vi "InMotion.vi"(0 "System no.":i32, 2 "Axes to check":string[](array[string]), 5 "error in (no error)":errorcluster, 9 "With status bit polling?":bool) -> (14 "InMotion":bool, 16 "Motion Error":bool, 19 "error out":errorcluster)   [LabVIEW 2020]
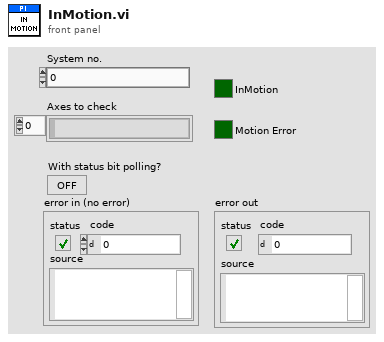
[diagram p1: front panel]
types:
  T1 = typedef "Syntax.ctl" = enum16{"GCS 1.0", "GCS 2.0", "GCS 3.0"}
  T2 = typedef "Status.ctl" = cluster{"Element":string, "Status bits":bool[]}
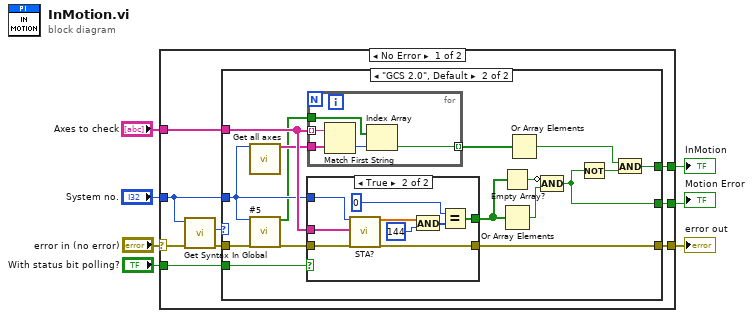
[diagram p0: block diagram]
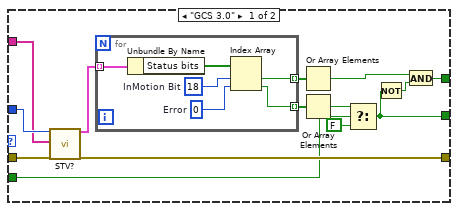
[diagram p2: hidden frame]
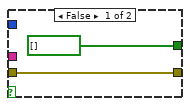
[diagram p3: hidden frame]
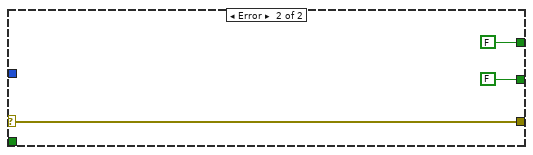
[diagram p4: hidden frame]
diagram:
  n1 = case shown="No Error" "error in (no error)" {
    selector: "error in (no error)" -> [w8 w71]
    tunnel: [w16 FALSE] -> w7
    tunnel: [w15 w71] -> w6
    tunnel: "With status bit polling?" -> [w14 _]
    tunnel: "Axes to check" -> [w13 _]
    tunnel: "System no." -> [w10 _]
    tunnel: [w9 FALSE] -> w2
    frame No Error {
      n2 = call "Get Syntax In Global.vi"("error in"=w8, "System no."=w10) -> ("error out"=w12:errorcluster, "Syntax"=w11:T1)  [unwired: 8 in]
      n3 = case shown="\"GCS 2.0\", Default" w11 {
        tunnel: w10 -> [w30 w47]
        tunnel: w12 -> [w29 w52]
        tunnel: [w28 w50] -> w15
        tunnel: [w19 w38] -> w16
        tunnel: w13 -> [w26 w49]
        tunnel: w14 -> [w21 w48]
        tunnel: [w17 w40] -> w9
        frame "GCS 3.0" {
          n4 = call "STV?.vi"("System no."=w30, "Status Type"=w26, "error in"=w29) -> ("Status Array"=w27:T2[], "error out"=w28:errorcluster)  [unwired: 15 in]
          n5 = for {
            tunnel: w27 -> [w36] mode=indexing
            tunnel: [w33] -> w25 mode=indexing
            tunnel: [w31] -> w23 mode=indexing
            w32 = 0  # Error
            w34 = 18  # InMotion Bit
            n6 = Unbundle By Name(w36) -> ("Status bits"=w35:bool[])
            n7 = Index Array(array=w35, index #1=w34, index #2=w32) -> (element #1=w33:bool, element #2=w31:bool)
          }
          n8 = Or Array Elements(Boolean array=w25) -> (logical OR=w24:bool)
          n9 = Or Array Elements(Boolean array=w23) -> (logical OR=w22:bool)
          n10 = Select(t=w22, s=w21, f=FALSE) -> (s? t:f=w17:bool)
          n11 = Not(x=w17) -> (.not. x?=w18:bool)
          n12 = And(x=w24, y=w18) -> (x .and. y?=w19:bool)
        }
        frame "GCS 2.0", Default {
          n13 = call "Get all axes.vi"("System no."=w47) -> ("Conn. Axes"=w46:string[])  [unwired: 18 out]
          n14 = call "#5.vi"("System no."=w47, "error in"=w52) -> ("Axis moving?"=w45:bool[], "error out"=w51:errorcluster)  [unwired: 16 out]
          n15 = case shown="True" w48 {
            tunnel: w51 -> [w53 w63]
            tunnel: [w53 w62] -> w50
            tunnel: w47 -> [_ w61]
            tunnel: w49 -> [_ w60]
            tunnel: [bool[] [] w56] -> w41
            frame False {
            }
            frame True {
              n16 = call "STA?.vi"("System no."=w61, "Axes to query"=w60, "error in"=w63) -> ("Axis status"=w58:dbl[], "error out"=w62:errorcluster)  [unwired: 2 in, 13 out]
              n17 = And(x=w58, y=u32 144) -> (x .and. y?=w55:i32[])
              n18 = Equal?(x=0 ("y"), y=w55) -> (x = y?=w56:bool[])
            }
          }
          n19 = for {
            tunnel: w46 -> [w67]
            tunnel: w49 -> [w68] mode=indexing
            tunnel: w45 -> [w66]
            tunnel: [w64] -> w44 mode=indexing
            n20 = Match First String(2:w67, 3:w68) -> (0:w65:i32)  [unwired: 1 out]
            n21 = Index Array(array=w66, index=w65) -> (element=w64:bool)
          }
          n22 = Empty Array?(array=w41) -> (empty?=w42:bool)
          n23 = Or Array Elements(Boolean array=w41) -> (logical OR=w43:bool)
          n24 = Or Array Elements(Boolean array=w44) -> (logical OR=w39:bool)
          n25 = Compound Arithmetic op=AND(invert w42, w43) -> (w40:bool)
          n26 = Not(x=w40) -> (.not. x?=w37:bool)
          n27 = And(x=w39, y=w37) -> (x .and. y?=w38:bool)
        }
      }
    }
    frame Error {
    }
  }
  "InMotion" <- w7
  "error out" <- w6
  "Motion Error" <- w2
